vi "Calculate Optimal Timebucket.vi"(9 "span (s)":dbl, 10 "max points":i32, 11 "Time Bucket in":T1) -> (3 "Time Bucket out":T1)   [LabVIEW 2019, in "Database Viewer.lvclass"]
uses:
  Database Viewer.lvclass
  typedefs/Time Bucket--enum.ctl
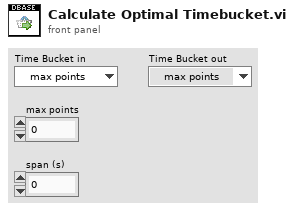
[diagram p1: front panel]
types:
  T1 = typedef "Database Viewer.lvclass/Time Bucket--enum.ctl" = enum16{"max points", "automatic", "1 second", "10 seconds", "1 minute", "10 minutes", "1 hour", "10 hours", "1 day", "10 days", "1 month"}
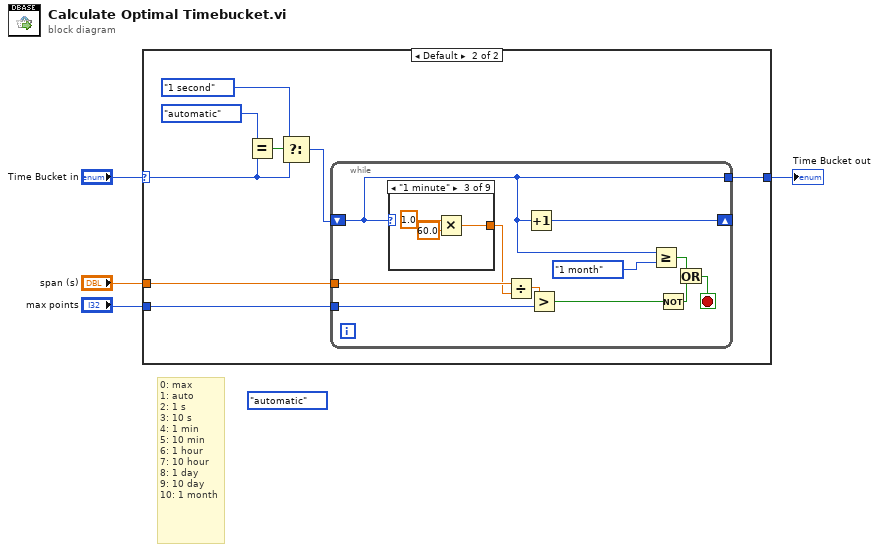
[diagram p0: block diagram]
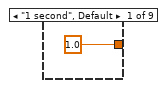
[diagram p3: hidden frame]
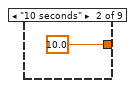
[diagram p4: hidden frame]
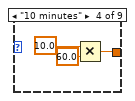
[diagram p5: hidden frame]
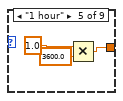
[diagram p6: hidden frame]
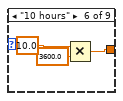
[diagram p7: hidden frame]
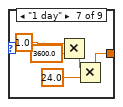
[diagram p8: hidden frame]
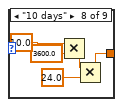
[diagram p9: hidden frame]
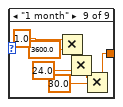
[diagram p10: hidden frame]
diagram:
  (unwired) Time_Bucket--enum."automatic" ("Time Bucket")
  # "0: max\n1: auto\n2: 1 s\n3: 10 s\n4: 1 min\n5: 10 min\n6: 1 hour\n7: 10 hour\n8: 1 day\n9: 10 day\n10: 1 month"
  n1 = case shown="Default" "Time Bucket in" {
    selector: "Time Bucket in" -> [w5 w6]
    tunnel: "max points" -> [_ w13]
    tunnel: [w5 w12] -> w3
    tunnel: "span (s)" -> [_ w11]
    frame "max points" {
    }
    frame Default {
      n2 = Equal?(x=Time_Bucket--enum."automatic" ("Time Bucket in"), y=w6) -> (x = y?=w9:bool)
      n3 = Select(t=Time_Bucket--enum."1 second" ("Time Bucket in"), s=w9, f=w6) -> (s? t:f=w7:T1)
      n4 = while {
        shift-right: [w24] -> _
        shift-left: w7 -> [w15]
        tunnel: w11 -> [w23]
        tunnel: [w15] -> w12
        tunnel: w13 -> [w16]
        stop <- w17 stop-if-true
        n5 = case shown="\"1 minute\"" w15 {
          tunnel: [1.0 10.0 w27 w30 w33 w36 w39 w44 w50] -> w22
          frame "1 second", Default {
          }
          frame "10 seconds" {
          }
          frame "1 minute" {
            n6 = Multiply(x=1.0, y=60.0) -> (x*y=w27:dbl)
          }
          frame "10 minutes" {
            n7 = Multiply(x=10.0, y=60.0) -> (x*y=w30:dbl)
          }
          frame "1 hour" {
            n8 = Multiply(x=1.0, y=3600.0) -> (x*y=w33:dbl)
          }
          frame "10 hours" {
            n9 = Multiply(x=10.0, y=3600.0) -> (x*y=w36:dbl)
          }
          frame "1 day" {
            n10 = Multiply(x=1.0, y=3600.0) -> (x*y=w41:dbl)
            n11 = Multiply(x=w41, y=24.0) -> (x*y=w39:dbl)
          }
          frame "10 days" {
            n12 = Multiply(x=10.0, y=3600.0) -> (x*y=w46:dbl)
            n13 = Multiply(x=w46, y=24.0) -> (x*y=w44:dbl)
          }
          frame "1 month" {
            n14 = Multiply(x=1.0, y=3600.0) -> (x*y=w53:dbl)
            n15 = Multiply(x=w53, y=24.0) -> (x*y=w51:dbl)
            n16 = Multiply(x=w51, y=30.0) -> (x*y=w50:dbl)
          }
        }
        n17 = Divide(x=w23, y=w22) -> (x/y=w21:dbl)
        n18 = Increment(x=w15) -> (x+1=w24:T1)
        n19 = Greater?(x=w21, y=w16) -> (0:w20:bool)
        n20 = Greater Or Equal?(x=w15, y=Time_Bucket--enum."1 month" ("Time Bucket in")) -> (x >= y?=w19:bool)
        n21 = Not(x=w20) -> (.not. x?=w18:bool)
        n22 = Or(x=w19, y=w18) -> (x .or. y?=w17:bool)
      }
    }
  }
  "Time Bucket out" <- w3
